vi "Max Bin Detection.vi"(0 "FFT Array":dbl[](array[numeric]), 2 "Init Discard Bins":i32=10, 3 "Last Discard Bins":i32=255) -> (14 "Prev Max Bin":i32, 15 "Max Bin":i32, 16 "Succ Max Bin":i32, 17 "Prev Max Amp":dbl, 18 "Max Amp":dbl, 19 "Succ Max Amp":dbl)   [LabVIEW 2014]
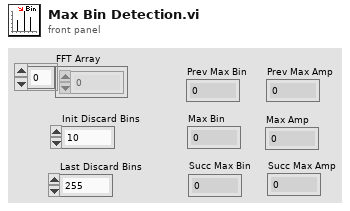
[diagram p1: front panel]
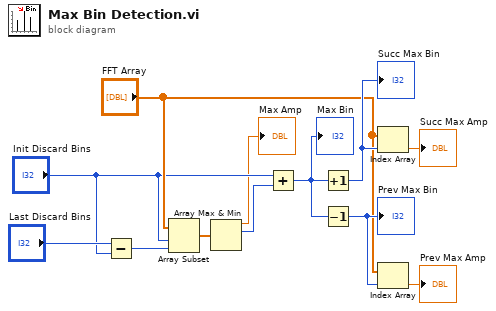
[diagram p0: block diagram]
diagram:
  n1 = Subtract(x="Last Discard Bins", y="Init Discard Bins") -> (x-y=w4:i32)
  n2 = Array Subset(array="FFT Array", index="Init Discard Bins", length=w4) -> (w12:dbl[])
  n3 = Array Max & Min(array=w12) -> (max value=→"Max Amp":dbl, max index (indices)=w11:i32)  [unwired: 2 out]
  n4 = Add(x="Init Discard Bins", y=w11) -> (x+y=w9:i32)
  "Max Bin" <- w9
  n5 = Increment(x=w9) -> (x+1=w10:i32)
  "Succ Max Bin" <- w10
  n6 = Decrement(x=w9) -> (x-1=w8:i32)
  "Prev Max Bin" <- w8
  n7 = Index Array(array="FFT Array", index=w10) -> (element=→"Succ Max Amp":dbl)
  n8 = Index Array(array="FFT Array", index=w8) -> (element=→"Prev Max Amp":dbl)
